vi "set_wavelength.vi"(8 "error in (no error)":errorcluster, 10 "wavelength in":dbl[unit], 11 "LightSourceAN191011Chameleon in":refnum<class "LightSourceAN191011Chameleon.lvclass">) -> (0 "error out":errorcluster, 3 "LightSourceAN191011Chameleon out":refnum<class "LightSourceAN191011Chameleon.lvclass">)   [LabVIEW 2010, in "LightSourceAN191011Chameleon.lvclass"]
uses:
  LightSourceAN191011Chameleon.lvclass
  LightSourceAN191011Chameleon.lvclass/LightSourceAN191011Chameleon.ctl
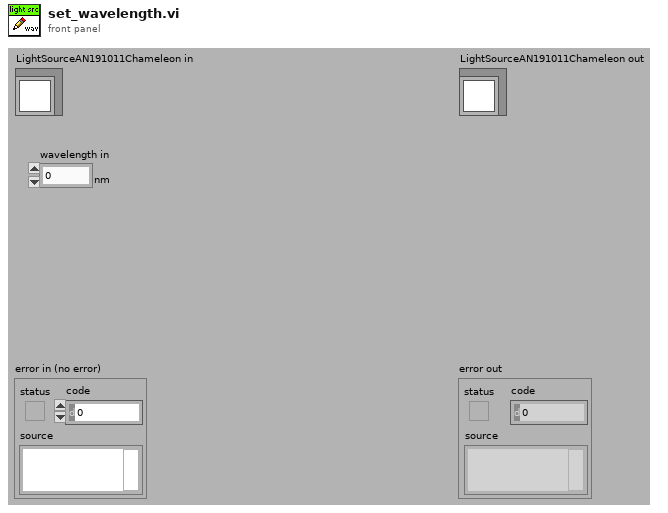
[diagram p1: front panel]
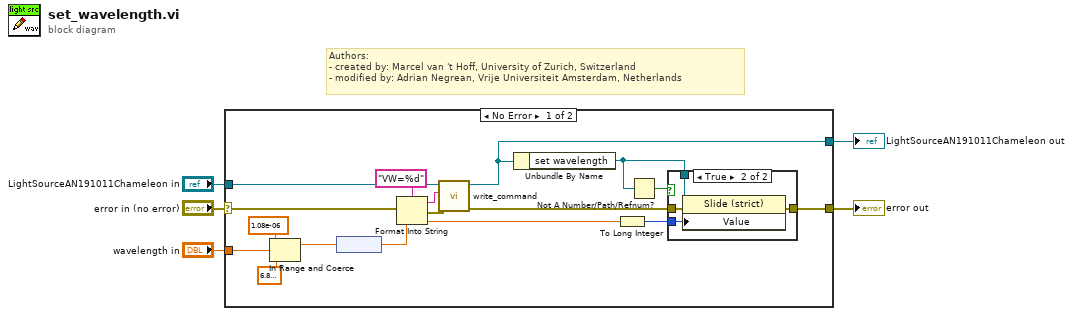
[diagram p0: block diagram]
diagram:
  # "Authors: \n- created by: Marcel van 't Hoff, University of Zurich, Switzerland\n- modified by: Adrian Negrean, Vrije Universiteit Amsterdam, Netherlands"
  n1 = case shown="No Error" "error in (no error)" {
    selector: "error in (no error)" -> [w17 w28]
    tunnel: [w13 w28] -> w4
    tunnel: [w15 w27] -> w2
    tunnel: "LightSourceAN191011Chameleon in" -> [w19 w27]
    tunnel: "wavelength in" -> [w21 _]
    frame No Error {
      n2 = In Range and Coerce(upper limit=dbl[unit] 1.08e-06, x=w21, lower limit=dbl[unit] 6.800000000000001e-07) -> (coerced(x)=w8:dbl[unit])  [unwired: 1 out]
      n3 = node(w8) -> (w6:dbl)
      n4 = Format Into String(format string="VW=%d", error in=w17, w6) -> (resulting string=w18:string, error out=w16:errorcluster)  [unwired: 1 in]
      n5 = call-dynamic "write_command.vi"("error in (no error)"=w16, "string to write"=w18, "LightSourceAN191011Chameleon in"=w19) -> ("error out"=w14:errorcluster, "LightSourceAN191011Chameleon out"=w15:refnum<class "LightSourceAN191011Chameleon.lvclass">)  [unwired: 6 in, 1 out]
      n6 = Unbundle By Name(w15) -> ("set wavelength"=w12:refnum<vi>)
      n7 = To Long Integer(number=w6) -> (32bit integer=w10:i32)
      n8 = Not A Number/Path/Refnum?(number/path/refnum=w12) -> (NaN/Path/Refnum?=w11:bool)
      n9 = case shown="True" w11 {
        tunnel: w12 -> [_ w26]
        tunnel: w14 -> [w22 w25]
        tunnel: [w22 w24] -> w13
        tunnel: w10 -> [_ w23]
        frame False {
        }
        frame True {
          n10 = property on="Property Node" class="Slide (strict)"(reference=w26, error in=w25, "Value"=w23) -> (error out=w24:errorcluster)  [unwired: 1 out]
        }
      }
    }
    frame Error {
    }
  }
  "error out" <- w4
  "LightSourceAN191011Chameleon out" <- w2
